vi "Write to List.vi"(9 "Publication Time":timestamp, 10 "Value to Publish":variant, 11 "Topic in":refnum<class "Topic.lvclass">) -> (3 "Topic out":refnum<class "Topic.lvclass">)   [LabVIEW 2017, in "Mediator.lvlib" / "Topic.lvclass"]
uses:
  Topic.lvclass
  Topic.lvclass/Topic.ctl
  IMediator/ISubscriptionPolicy/ISubscriptionPolicy Reference.ctl
  IMediator/ISubscriptionPolicy/ISubscriptionPolicy.lvclass
  IMediator/ISubscriptionPolicy/ISubscriptionPolicy.lvclass/ISubscriptionPolicy.ctl
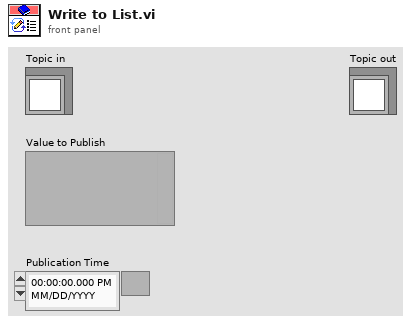
[diagram p1: front panel]
types:
  T1 = typedef "IMediator.lvlib/ISubscriptionPolicy.lvclass/ISubscriptionPolicy Reference.ctl" = refnum<data-value>
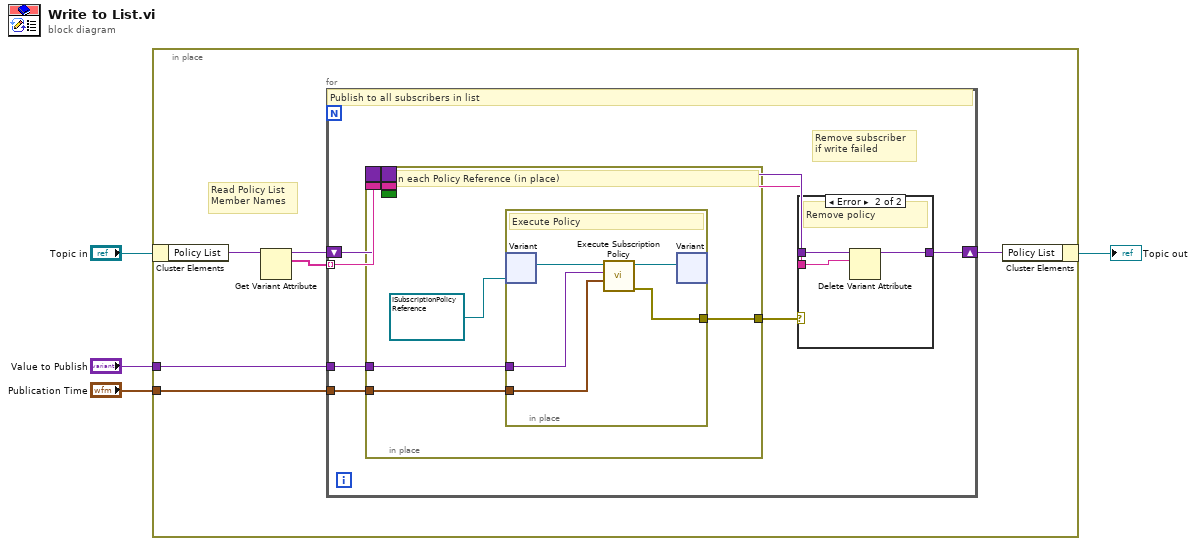
[diagram p0: block diagram]
diagram:
  n1 = in-place {
    in-place-border: "Publication Time" -> [w10]
    in-place-border: "Value to Publish" -> [w9]
    # "Read Policy List\nMember Names"
    n2 = in-place-cluster #1("Topic in") -> ("Policy List"=w6:variant)
    n3 = Get Variant Attribute(Variant=w6) -> (duplicate Variant=w7:variant, names=w8:string[])  [unwired: 3 in, 2 out]
    n4 = for {
      tunnel: w9 -> [w18]
      tunnel: w10 -> [w17]
      shift-right: [w13] -> w5
      shift-left: w7 -> [w15]
      tunnel: w8 -> [w16] mode=indexing
      # "Remove subscriber\nif write failed"
      # "Publish to all subscribers in list"
      n5 = in-place {
        in-place-border: [w23] -> w11
        in-place-border: w18 -> [w28]
        in-place-border: w17 -> [w27]
        border: w15 -> [_]
        border: w16 -> [_]
        border: [_] -> w14
        border: [_] -> w12
        border: _ -> [_]
        # "Obtain each Policy Reference (in place)"
        n6 = in-place {
          in-place-border: [w33] -> w23
          in-place-border: w28 -> [w32]
          in-place-border: w27 -> [w31]
          # "Execute Policy"
          n7 = in-place-variant #2(w26, T1 refnum ("Subscription Policy")) -> (w30:T1)  [unwired: 1 out]
          n8 = call "Execute Subscription Policy.vi"("Publish Time"=w31, "New Topic Value"=w32, "Subscription Policy"=w30) -> ("error out (Unsubscribe?)"=w33:errorcluster, "Subscription Policy Out"=w29:T1)  [unwired: 7 in]
          n9 = in-place-variant #2(w29) -> (w24:variant)  [unwired: 1 out]
        }
      }
      n10 = case shown="Error" w11 {
        tunnel: w14 -> [w19 w22]
        tunnel: [w19 w21] -> w13
        tunnel: w12 -> [_ w20]
        frame No Error {
          # "Write OK"
        }
        frame Error {
          # "Remove policy"
          n11 = Delete Variant Attribute(6:w20, 7:w22) -> (3:w21:variant)  [unwired: 1 in, 2 out]
        }
      }
    }
    n12 = in-place-cluster #1("Policy List"=w5) -> (→"Topic out":refnum<class "Topic.lvclass">)
  }
